vi "runCI2_tt.vi"   [LabVIEW 2013]
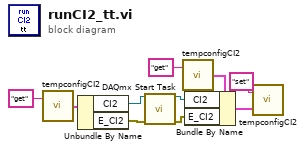
[diagram p0: block diagram]
diagram:
  n1 = call "tempconfigCI2.vi"("command"="get") -> ("Temp Config out"=w3:cluster{"CI2":refnum<k21>, "E_CI2":errorcluster})  [unwired: 1 in]
  n2 = Unbundle By Name(w3) -> ("CI2"=w2:refnum<k21>, "E_CI2"=w1:errorcluster)
  n3 = call <vilib>:"DAQmx Start Task.vi"("task/channels in"=w2, "error in"=w1) -> ("task out"=w5:refnum<k21>, "error out"=w6:errorcluster)  [unwired: 12 in]
  n4 = call "tempconfigCI2.vi"("command"="get") -> ("Temp Config out"=w7:cluster{"CI2":refnum<k21>, "E_CI2":errorcluster})  [unwired: 1 in]
  n5 = Bundle By Name(cluster=w7, "CI2"=w5, "E_CI2"=w6) -> (w10:cluster{"CI2":refnum<k21>, "E_CI2":errorcluster})
  n6 = call "tempconfigCI2.vi"("Temp Config in"=w10, "command"="set") -> ()  [unwired: 1 out]
